vi "LatchRefSelector.vi"() -> ()   [LabVIEW 2014, in "LatchLib.lvlib"]
uses:
  LatchLib.lvlib
  LatchRefs.ctl
panel:
  out "String":string="FrontRightIntakeMotor"
  in  "Enum":T1
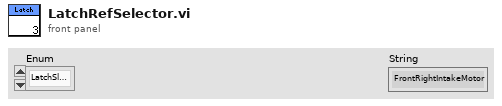
[diagram p1: front panel]
types:
  T1 = typedef "LatchLib.lvlib/LatchRefs.ctl" = enum16{"LatchSloenoid", "ContainerSolenoid"}
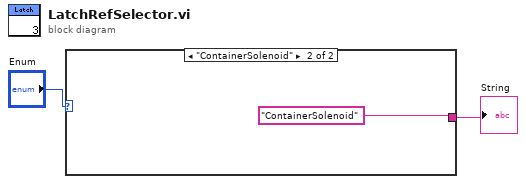
[diagram p0: block diagram]
diagram:
  n1 = case shown="\"ContainerSolenoid\"" "Enum" {
    tunnel: [_ "ContainerSolenoid"] -> w1
    frame "LatchSloenoid", Default {
    }
    frame "ContainerSolenoid" {
    }
  }
  "String" <- w1
